vi "1A Helper - wait for $ on serial.vi"(7 "error in (no error)":errorcluster, 9 "# of tries (100)":i32=100, 10 "Serial Refnum in":refnum<visa-resource-name>) -> (0 "error out":errorcluster, 2 "Succeeded":bool, 3 "Serial Refnum out":refnum<visa-resource-name>)   [LabVIEW 2011]
doc: "Listens to up to 100 characters on the given serial port and returns when it recieves a dollar sign ($). If a $ is not recieved in 100 tries or if the E-Stop is hit, will return an appropriate boolean."
uses:
  2-Think/2 Globals/2 Global.vi
panel:
  out "Try count":i32
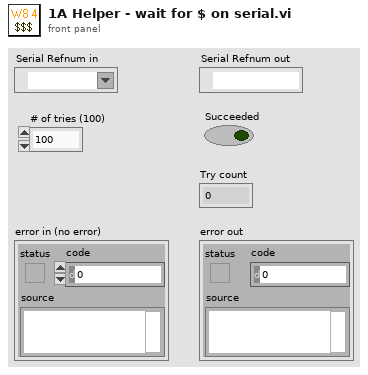
[diagram p1: front panel]
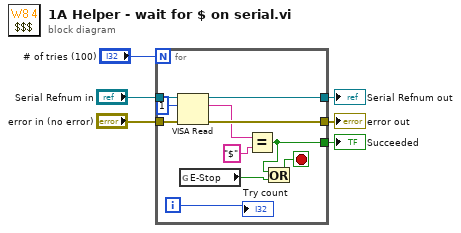
[diagram p0: block diagram]
diagram:
  n1 = for {
    N: "# of tries (100)" -> [_]
    tunnel: [w17] -> w1
    tunnel: "Serial Refnum in" -> [w16]
    tunnel: "error in (no error)" -> [w15]
    tunnel: [w14] -> w4
    tunnel: [w9] -> w5
    i -> [w7]
    stop <- w10 stop-if-true
    n2 = VISA Read(VISA resource name=w16, byte count=u32 1, error in (no error)=w15) -> (VISA resource name out=w17:refnum<visa-resource-name>, read buffer=w12:string, error out=w14:errorcluster)  [unwired: 1 out]
    n3 = global read "2 Global.vi" "E-Stop"() -> (w8:bool)
    n4 = Equal? ("wait for a $, which indicates\nsensor initialized")(x=w12, y="$" ("x")) -> (x = y?=w9:bool)
    n5 = Or(x=w9, y=w8) -> (x .or. y?=w10:bool)
    "Try count" <- w7
  }
  "Succeeded" <- w5
  "error out" <- w4
  "Serial Refnum out" <- w1
